vi "VA Hatch Test.vi"(7 "error in":errorcluster) -> (27 "error out":errorcluster)   [LabVIEW 2018]
uses:
  <vilib>/vision/NI_Vision_Development_Module.lvlib
panel:
  out "Image Out":T1(plugin-control)
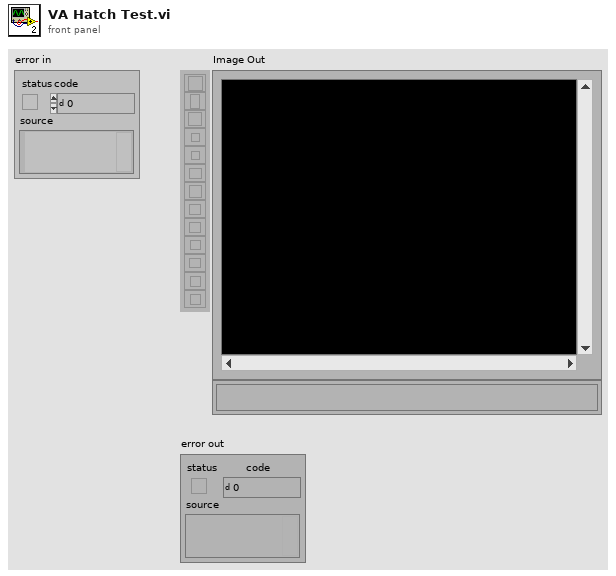
[diagram p1: front panel]
types:
  T1 = typedef "IMAQ Image.ctl" = refnum<image>
  T2 = cluster{"Measurement Parameter":i32, "Range Lower Value":dbl, "Range Upper Value":dbl, "Range":bool, "Measurement Type":bool}[]
  T3 = typedef "Image Type" = u32
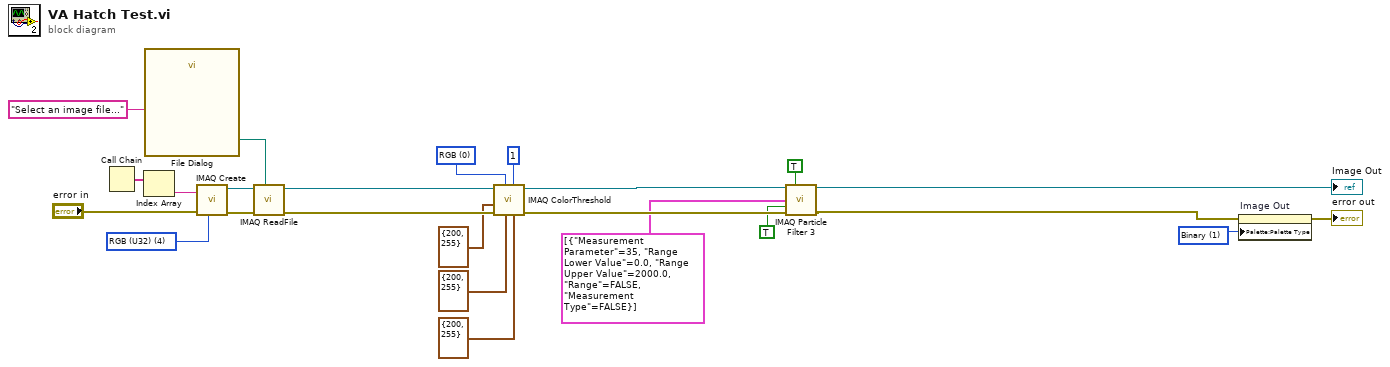
[diagram p0: block diagram]
diagram:
  w3 = u32 1 items=["Grayscale", "Binary", "Gradient", "Rainbow", "Temperature", "User Defined", "Binary 16 Bit", "Gradient 16 Bit", "Rainbow 16 Bit", "Temperature 16 Bit", "User Defined 16 Bit"] ("Palette Type")
  w14 = u16 0 items=["RGB", "HSL", "HSV", "HSI"] ("Color Mode")
  w16 = T3 4 items=["Grayscale (U8)", "Grayscale (I16)", "Grayscale (SGL)", "Complex (CSG)", "RGB (U32)", "HSL (U32)", "RGB (U64)", "Grayscale (U16)"] ("Image Type")
  n1 = Call Chain() -> (call chain=w20:string[])
  n2 = Index Array(array=w20) -> (element=w19:string)  [unwired: 1 in]
  n3 = call "File Dialog"("prompt"="Select an image file...") -> ("selected path"=w17:path)  [unwired: 6 in, 8 out]
  n4 = call "IMAQ Create"("Image Name"=w19, "Image Type"=w16, "error in (no error)"="error in") -> ("New Image"=w23:T1, "error out"=w22:errorcluster)  [unwired: 1 in, 1 out]
  n5 = call "IMAQ ReadFile"("File Path"=w17, "error in (no error)"=w22, "Image"=w23) -> ("error out"=w24:errorcluster, "Image Out"=w10:T1)  [unwired: 2 in, 5 out]
  n6 = call "IMAQ ColorThreshold"("Blue or Luma or Val or Inten Range"=cluster{"Lower value":i32, "Upper value":i32} {"Lower value"=200, "Upper value"=255}, "Replace Value"=1, "Green or Sat Range"=cluster{"Lower value":i32, "Upper value":i32} {"Lower value"=200, "Upper value"=255}, "Color Mode"=w14, "error in (no error)"=w24, "Red or Hue Range"=cluster{"Lower value":i32, "Upper value":i32} {"Lower value"=200, "Upper value"=255}, "Image Src"=w10) -> ("error out"=w9:errorcluster, "Image Dst Out"=w6:T1)  [unwired: 1 in, 2 out]
  n7 = call "IMAQ Particle Filter 3"("Image Src"=w6, "Connectivity 4/8 (8)"=TRUE, "Selection Values"=T2 [{"Measurement Parameter"=35, "Range Lower Value"=0.0, "Range Upper Value"=2000.0, "Range"=FALSE, "Measurement Type"=FALSE}], "Keep/Remove Particles (F)"=TRUE ("Keep/Remove Particles"), "error in (no error)"=w9) -> ("Image Dst Out"=→"Image Out":T1, "error out"=w2:errorcluster)  [unwired: 4 in, 5 out]
  n8 = property on="Image Out" class="ImageControl"(error in=w2, "Palette:Palette Type"=w3) -> (error out=→"error out":errorcluster)  [unwired: 1 in, 1 out]
